vi "Resistor card.vi"(8 "error in (no error)":errorcluster, 11 "Node Ptr":T4 format="%.0x") -> (0 "error out":errorcluster)   [LabVIEW 2014, in "SLSC configuration System Explorer.lvlib"]
uses:
  SLSC configuration System Explorer.lvlib
  <vilib>/NI Veristand/Custom Device API/Custom Device Item Ref.ctl
  Type Defs/Card Position.ctl
  Shared/SPI Utility/Slot #.ctl
  Shared/Resistor Board/Resistance.ctl
  Shared/Constants.vi
  <vilib>/NI Veristand/Custom Device API/Get Item Property (U16).vi
  <vilib>/NI Veristand/Custom Device API/Custom Device API.lvlib
  Shared/SLSC configuration Shared.lvlib
panel:
  in  "Resistance 8 (Ohms)":T1=5.12555 min=2.0 max=8193.875 format="%#_7g"
  in  "Resistance 7 (Ohms)":T1=5.12555 min=2.0 max=8193.875 format="%#_7g"
  in  "Resistance 6 (Ohms)":T1=5.12555 min=2.0 max=8193.875 format="%#_7g"
  in  "Resistance 5 (Ohms)":T1=5.12555 min=2.0 max=8193.875 format="%#_7g"
  in  "Header 8":cluster{"Section Name":string}={"Section Name"="Bank 7 Settings"}
  in  "Header 7":cluster{"Section Name":string}={"Section Name"="Bank 6 Settings"}
  in  "Header 6":cluster{"Section Name":string}={"Section Name"="Bank 5 Settings"}
  in  "Header 5":cluster{"Section Name":string}={"Section Name"="Bank 4 Settings"}
  in  "Resistance 4 (Ohms)":T1=5.12555 min=2.0 max=8193.875 format="%#_7g"
  in  "Resistance 3 (Ohms)":T1=5.12555 min=2.0 max=8193.875 format="%#_7g"
  in  "Resistance 2 (Ohms)":T1=5.12555 min=2.0 max=8193.875 format="%#_7g"
  in  "Resistance 1 (Ohms)":T1=5.12555 min=2.0 max=8193.875 format="%#_7g"
  in  "Header 4":cluster{"Section Name":string}={"Section Name"="Bank 3 Settings"}
  in  "Header 2":cluster{"Section Name":string}={"Section Name"="Bank 2 Settings"}
  in  "Header 3":cluster{"Section Name":string}={"Section Name"="Bank 1 Settings"}
  in  "Card Position":T2 {"Slot #" max=15}
  in  "Header 2":cluster{"Section Name":string}={"Section Name"="Bank 0 Settings"}
  in  "Header":cluster{"Section Name":string}={"Section Name"="Resistor Card Settings"}
  in  "Description":string
  in  "Name":string
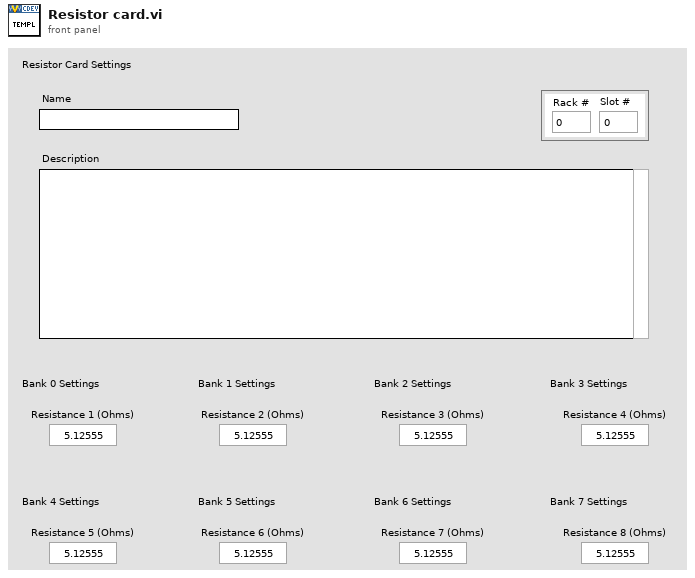
[diagram p1: front panel]
types:
  T1 = typedef "SLSC configuration Shared.lvlib/Resistance.ctl" = dbl
  T2 = typedef "SLSC configuration Shared.lvlib/Card Position.ctl" = cluster{"Rack #":u8, "Slot #":T3}
  T3 = typedef "SLSC configuration Shared.lvlib/Slot #.ctl" = u8
  T4 = typedef "Custom Device API.lvlib/Custom Device Item Ref.ctl" = u64
  T5 = typedef "Custom Device API.lvlib/Custom Device Item Info.ctl" = cluster{"Name":string, "Is Channel":bool, "GUID":string, "Is Waveform":bool}
  T6 = typedef "Custom Device API.lvlib/Custom Device Commands.ctl" = enum16{"Default", "Item renamed", "Shutdown", "Dynamic button pressed"}
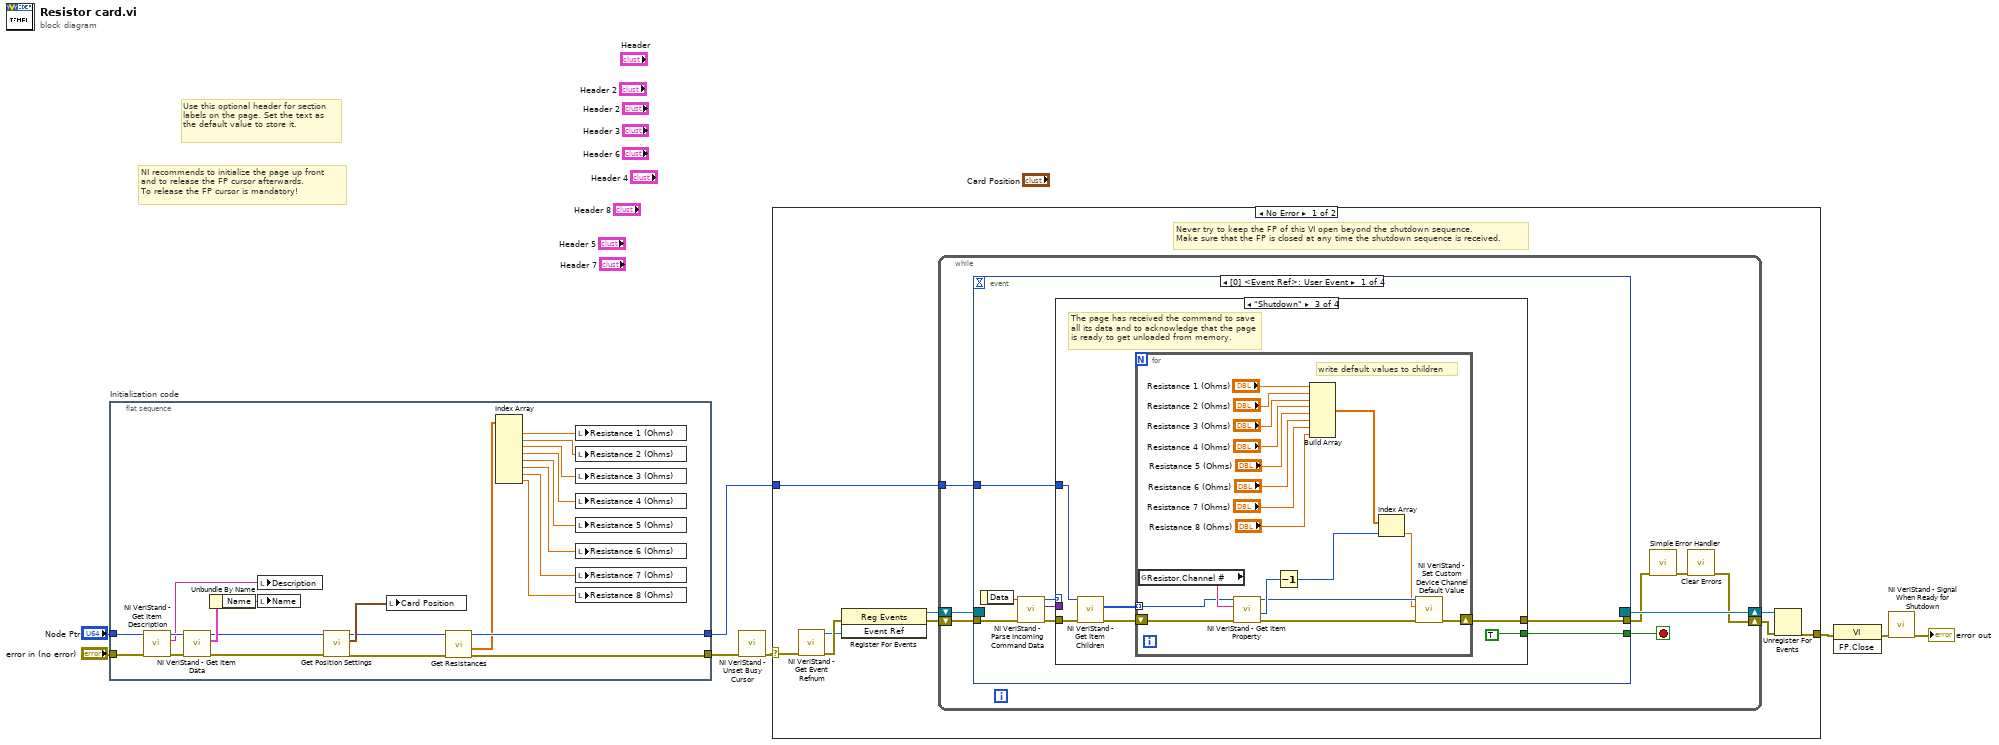
[diagram p0: block diagram]
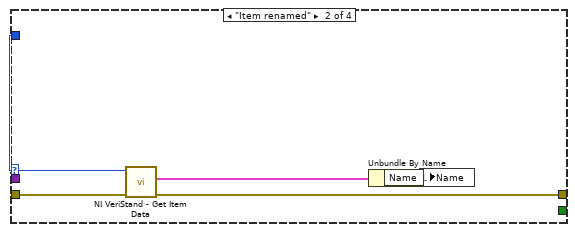
[diagram p3: hidden frame]
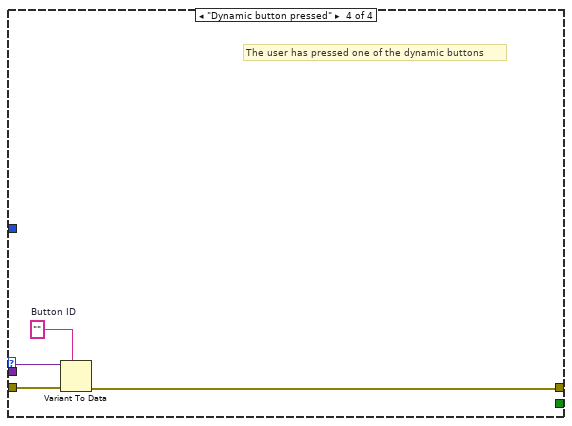
[diagram p4: hidden frame]
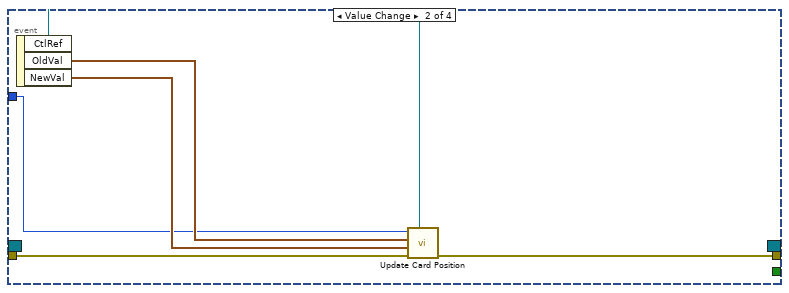
[diagram p5: hidden frame]
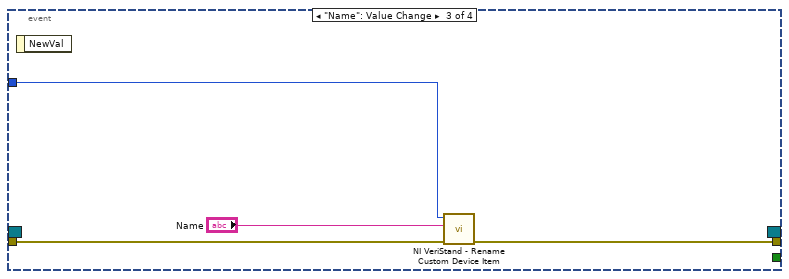
[diagram p6: hidden frame]
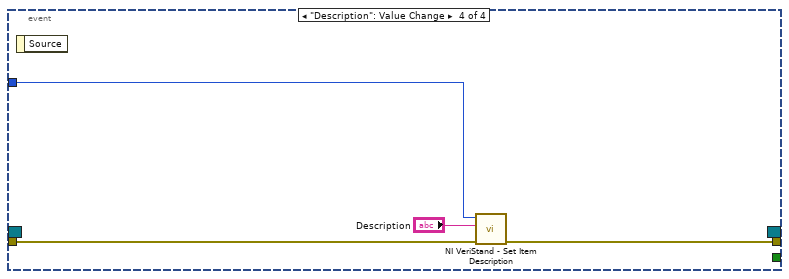
[diagram p7: hidden frame]
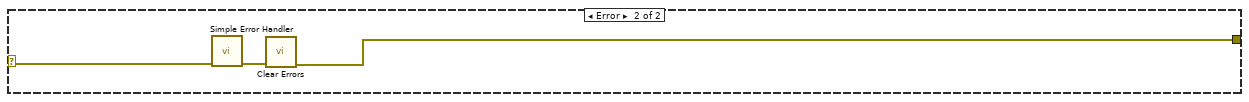
[diagram p8: hidden frame]
diagram:
  # "Use this optional header for section labels on the page. Set the text as the default value to store it."
  # "NI recommends to initialize the page up front\nand to release the FP cursor afterwards.\nTo release the FP cursor is mandatory!"
  n1 = flat-sequence "Initialization code" {
    tunnel: "error in (no error)" -> [w30]
    tunnel: "Node Ptr" -> [w29]
    tunnel: [w19] -> w4
    tunnel: [w20] -> w1
    frame #0 {
      n2 = call <vilib>:"NI VeriStand - Get Item Description.vi"("error in (no error)"=w30, "Item Ref in"=w29) -> ("error out"=w27:errorcluster, "Description"=w28:string, "Item Ref out"=w31:T4)  [unwired: 7 out]
      n3 = call <vilib>:"NI VeriStand - Get Item Data.vi"("error in (no error)"=w27, "Item Ref in"=w31) -> ("error out"=w24:errorcluster, "Item Info"=w26:T5, "Item Ref out"=w23:T4)  [unwired: 7 out]
      n4 = Unbundle By Name(w26) -> ("Name"=w25:string)
      n5 = local write "Description"(w28) -> ()
      n6 = local write "Name"(w25) -> ()
      n7 = call "Get Position Settings.vi"("error in (no error)"=w24, "Item Ref in"=w23) -> ("error out"=w18:errorcluster, "Card Position"=w22:T2, "Item Ref out"=w21:T4)  [unwired: 7 in]
      n8 = local write "Card Position"(w22) -> ()
      n9 = call "Get Resistances.vi"("error in (no error)"=w18, "Item Ref in"=w21) -> ("error out"=w19:errorcluster, "Resistor Resistances"=w17:T1[], "Item Ref out"=w20:T4)  [unwired: 6 in, 1 out]
      n10 = Index Array(array=w17) -> (element #1=w16:T1, element #2=w15:T1, element #3=w14:T1, element #4=w13:T1, element #5=w12:T1, element #6=w11:T1, element #7=w10:T1, element #8=w9:T1)  [unwired: 8 in]
      n11 = local write "Resistance 1 (Ohms)"(w16) -> ()
      n12 = local write "Resistance 2 (Ohms)"(w15) -> ()
      n13 = local write "Resistance 3 (Ohms)"(w14) -> ()
      n14 = local write "Resistance 4 (Ohms)"(w13) -> ()
      n15 = local write "Resistance 5 (Ohms)"(w12) -> ()
      n16 = local write "Resistance 6 (Ohms)"(w11) -> ()
      n17 = local write "Resistance 7 (Ohms)"(w10) -> ()
      n18 = local write "Resistance 8 (Ohms)"(w9) -> ()
    }
  }
  n19 = call <vilib>:"NI VeriStand - Unset Busy Cursor.vi"("error in (no error)"=w4) -> ("error out"=w3:errorcluster)  [unwired: 10 out]
  n20 = case shown="No Error" w3 {
    selector: w3 -> [w32 w107]
    tunnel: [w37 w105] -> w8
    tunnel: w1 -> [w33 _]
    frame No Error {
      # "Never try to keep the FP of this VI open beyond the shutdown sequence.\nMake sure that the FP is closed at any time the shutdown sequence is received."
      n21 = call <vilib>:"NI VeriStand - Get Event Refnum.vi"("error in (no error)"=w32) -> ("error out"=w40:errorcluster, "Event Ref"=w36:refnum<user-event>)  [unwired: 9 out]
      n22 = register-events(error in=w40, w36) -> (reference out=w34:refnum<event-registration>, error out=w35:errorcluster)  [unwired: 1 in]
      n23 = while {
        tunnel: w33 -> [w44]
        shift-right: [w41] -> w38
        shift-left: w35 -> [w47]
        shift-right: [w48] -> w39
        shift-left: w34 -> [w46]
        stop <- w45 stop-if-true
        n24 = event shown="[0] <Event Ref>: User Event" {
          selector: w46 -> [_ _ _ _]
          dyn-events: [_ _ _ _] -> w48
          timeout: _ -> [_ _ _ _]
          tunnel: w47 -> [w56 w96 w100 w103]
          tunnel: [w52 _ _ _] -> w45
          tunnel: [w51 w95 w99 w102] -> w43
          tunnel: w44 -> [w50 w92 w98 w104]
          event User Event {
            n25 = event-data() -> ("Data"=w55:string)  [unwired: 1 out]
            n26 = call <vilib>:"NI VeriStand - Parse Incoming Command Data.vi"("error in (no error)"=w56, "Incoming data"=w55) -> ("error out"=w54:errorcluster, "Outgoing data"=w49:variant, "Action"=w53:T6)  [unwired: 7 out]
            n27 = case shown="\"Shutdown\"" w53 {
              tunnel: w54 -> [w57 w62 w67 w90]
              tunnel: [_ _ TRUE _] -> w52
              tunnel: [w57 w59 w63 w87] -> w51
              tunnel: w50 -> [_ w61 w66 _]
              tunnel: w49 -> [_ _ _ w89]
              frame "Default", Default {
              }
              frame "Item renamed" {
                n28 = call <vilib>:"NI VeriStand - Get Item Data.vi"("error in (no error)"=w62, "Item Ref in"=w61) -> ("error out"=w59:errorcluster, "Item Info"=w60:T5)  [unwired: 8 out]
                n29 = Unbundle By Name(w60) -> ("Name"=w58:string)
                n30 = local write "Name"(w58) -> ()
              }
              frame "Shutdown" {
                # "The page has received the command to save all its data and to acknowledge that the page is ready to get unloaded from memory."
                n31 = call <vilib>:"NI VeriStand - Get Item Children.vi"("error in (no error)"=w67, "Item Ref in"=w66) -> ("error out"=w65:errorcluster, "Child Refs"=w64:T4[])  [unwired: 6 in, 2 out]
                n32 = for {
                  shift-right: [w78] -> w63
                  shift-left: w65 -> [w85]
                  tunnel: w64 -> [w83] mode=indexing
                  # "write default values to children"
                  n33 = global read "Constants.vi" "Resistor.Channel #"() -> (w86:string)
                  n34 = call-poly <vilib>:"NI VeriStand - Get Item Property.vi"("error in (no error)"=w85, "Property Name"=w86, "Item Ref in"=w83) -> ("error out"=w81:errorcluster, "Value"=w84:u16, "Item Ref out"=w80:T4)  [unwired: 5 in, 1 out]
                  n35 = Decrement(x=w84) -> (x-1=w82:u16)
                  n36 = Build Array("Resistance 1 (Ohms)", "Resistance 2 (Ohms)", "Resistance 3 (Ohms)", "Resistance 4 (Ohms)", "Resistance 5 (Ohms)", "Resistance 6 (Ohms)", "Resistance 7 (Ohms)", "Resistance 8 (Ohms)") -> (w69:T1[])
                  n37 = Index Array(array=w69, index=w82) -> (element=w79:T1)
                  n38 = call <vilib>:"NI VeriStand - Set Custom Device Channel Default Value.vi"("error in (no error)"=w81, "Default Value"=w79, "Channel Ref in"=w80) -> ("error out"=w78:errorcluster)  [unwired: 7 in, 1 out]
                }
              }
              frame "Dynamic button pressed" {
                w88 = ""  # Button ID
                # "The user has pressed one of the dynamic buttons"
                n39 = Variant To Data(error in=w90, type=w88, Variant=w89) -> (error out=w87:errorcluster)  [unwired: 1 out]
              }
            }
          }
          event Value Change {
            n40 = event-data() -> ("CtlRef"=w91:refnum<vi>, "OldVal"=w93:T2, "NewVal"=w94:T2)  [unwired: 1 out]
            n41 = call "Update Card Position.vi"("Card Position Ref"=w91, "error in (no error)"=w96, "NewVal"=w94, "OldVal"=w93, "Node Ptr in"=w92) -> ("error out"=w95:errorcluster)  [unwired: 6 in]
          }
          event "Name": Value Change {
            n42 = event-data() -> ()  [unwired: 2 out]
            n43 = call <vilib>:"NI VeriStand - Rename Custom Device Item.vi"("error in (no error)"=w100, "New Name"="Name", "Item Ref in"=w98) -> ("error out"=w99:errorcluster)  [unwired: 1 in, 7 out]
          }
          event "Description": Value Change {
            n44 = event-data() -> ()  [unwired: 2 out]
            n45 = call <vilib>:"NI VeriStand - Set Item Description.vi"("error in (no error)"=w103, "Description"="Description", "Item Ref in"=w104) -> ("error out"=w102:errorcluster)  [unwired: 8 out]
          }
        }
        n46 = call <vilib>:"Simple Error Handler.vi"("error in (no error)"=w43) -> ("error out"=w42:errorcluster)  [unwired: 1 in, 7 out]
        n47 = call <vilib>:"Clear Errors.vi"("error in (no error)"=w42) -> ("error out"=w41:errorcluster)  [unwired: 1 in, 5 out]
      }
      n48 = Unregister For Events(event registration refnum=w39, error in=w38) -> (error out=w37:errorcluster)
    }
    frame Error {
      n49 = call <vilib>:"Simple Error Handler.vi"("error in (no error)"=w107) -> ("error out"=w106:errorcluster)  [unwired: 1 in, 7 out]
      n50 = call <vilib>:"Clear Errors.vi"("error in (no error)"=w106) -> ("error out"=w105:errorcluster)  [unwired: 1 in, 5 out]
    }
  }
  n51 = invoke class="VI" method="FP.Close"(error in=w8) -> (error out=w7:errorcluster)  [unwired: 2 in, 2 out]
  n52 = call <vilib>:"NI VeriStand - Signal When Ready for Shutdown.vi"("error in (no error)"=w7) -> ("error out"=→"error out":errorcluster)  [unwired: 10 out]
